vi "Flow and Pressure Sensor V6.vi"() -> ()   [LabVIEW 2018]
uses:
  <vilib>/Utility/config.llb/Config Data RefNum.ctl
  <vilib>/Utility/sysdir.llb/System Directory Type.ctl
  Program Files/National Instruments/LabVIEW 2018/examples/Instrument IO/Serial/support/Serial - XON-XOFF Characters.ctl
  Program Files/National Instruments/LabVIEW 2018/examples/Instrument IO/Serial/support/Serial - ASCII Characters.ctl
  Program Files/National Instruments/LabVIEW 2018/examples/Instrument IO/Serial/support/Serial - Settings.ctl
  <vilib>/Utility/config.llb/Read Key (String).vi
  <vilib>/Utility/config.llb/Write Key (String).vi
  <vilib>/Utility/config.llb/NI_LVConfig.lvlib
panel:
  out "RPM":string
  in  "Pump Speed":dbl(slide) step=1.0 scale=0.0..1023.0 scale format="%#.2f"
  out "Pressure Output":string
  out "Flow Output":string
  out "Raw Data":string
  out "Pressure":dbl(graph)
  out "Flow":dbl(graph)
  out "error out":errorcluster
  out "queue":refnum<queue>
  out "Driver Status":errorcluster
  in  "Marker":string="start_marker"
  out "State":enum16{"Connect", "Acquire", "Standby"}(ring)=enum."Standby"
  in  "S4":dbl[](array[numeric])=[0.0, 0.0, 0.0, 0.0]
  in  "S3":dbl[](array[numeric])=[0.0, 0.0, 0.0, 0.0]
  in  "S2":dbl[](array[numeric])=[0.0, 0.0, 0.0, 0.0]
  in  "S1":dbl[](array[numeric])=[0.0, 0.0, 0.0, 0.0]
  out "System Path":path
  out "dStruct":string[](array[string])
  out "TDMS":refnum<k34>
  in  "Tab Control":enum32{"Connection", "Diagnostic"}(tab)
  in  "Record":bool
  in  "New File":bool
  in  "markerString":string
  in  "Folder":path
  in  "File Name":string="database"
  in  "VISA":refnum<visa-resource-name>="COM4"
  in  "EXIT":bool
  in  "Connect":bool
  in  "add marker":bool
  out "Latency:":dbl
  out "Terminal":string
  in  "Command Terminal":string
  out "Serial Settings:Number of Bytes at Serial Port":u32
  out "Device:":string
  out "Battery Voltage":dbl(slide) scale=3.2..4.2 scale format="%#_2g"
  out "Error Out":errorcluster
  out "Config File":T1
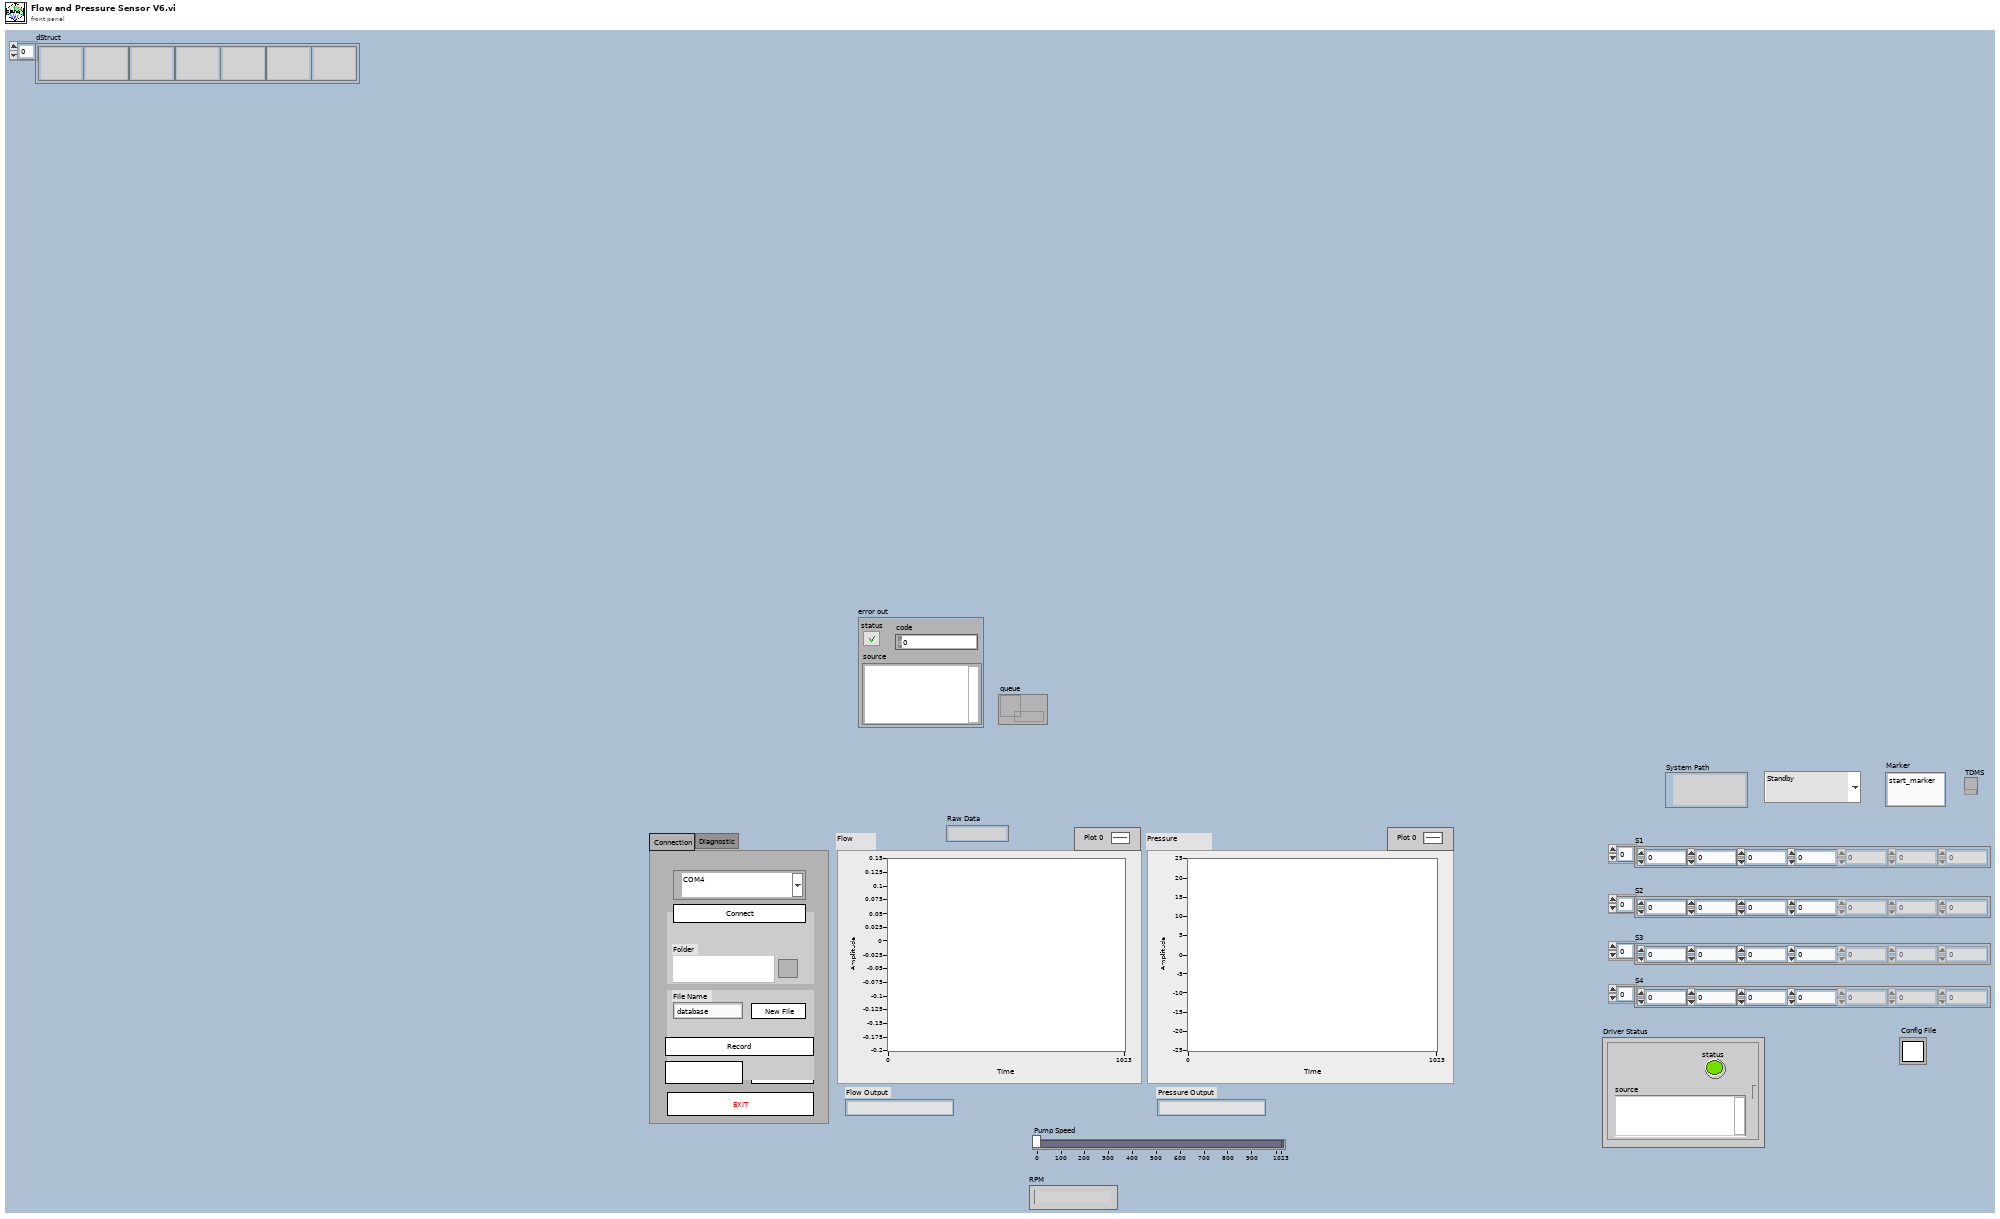
[diagram p1: front panel]
types:
  T1 = typedef "NI_LVConfig.lvlib/Config Data RefNum.ctl" = refnum<k1>
  T2 = cluster{"Dynamic Data Type":dynamicdata, string[]}
  T3 = typedef "System Directory Type.ctl" = i32
  T4 = typedef "Serial - Settings.ctl" = cluster{"baud rate":u32, "data bits":u16, "parity":enum16{"None", "Odd", "Even", "Mark", "Space"}, "stop bits":u16, "flow control":u16}
  T5 = typedef "Serial - XON-XOFF Characters.ctl" = cluster{"XON":T6, "XOFF":T6}
  T6 = typedef "Serial - ASCII Characters.ctl" = enum16{"NUL", "SOH", "STX", "ETX", "EOT", "ENQ", "ACK", "BEL", "BS", "HT", "LF", "VT", "FF", "CR", "SO", "SI", "DLE", "DC1", "DC2", "DC3", "DC4", "NAK", "SYN", "ETB", "CAN", "EM", "SUB", "ESC", "FS", "GS", "RS", "US", "SP", "!", "\"", "#", "$", "%", "&", "'", "(", ")", "*", "+", ",", "- (-)", ".", "/", "0", "1", "2", "3", "4", "5", "6", "7", "8", "9", ":", ";", "<", "=", ">", "?", "@", "A", "B", "C", "D", "E", "F", "G", "H", "I", "J", "K", "L", "M", "N", "O", "P", "Q", "R", "S", "T", "U", "V", "W", "X", "Y", "Z", "[", "\\", "]", "^", "_", "`", "a", "b", "c", "d", "e", "f", "g", "h", "i", "j", "k", "l", "m", "n", "o", "p", "q", "r", "s", "t", "u", "v", "w", "x", "y", "z", "{", "|", "}", "~"}
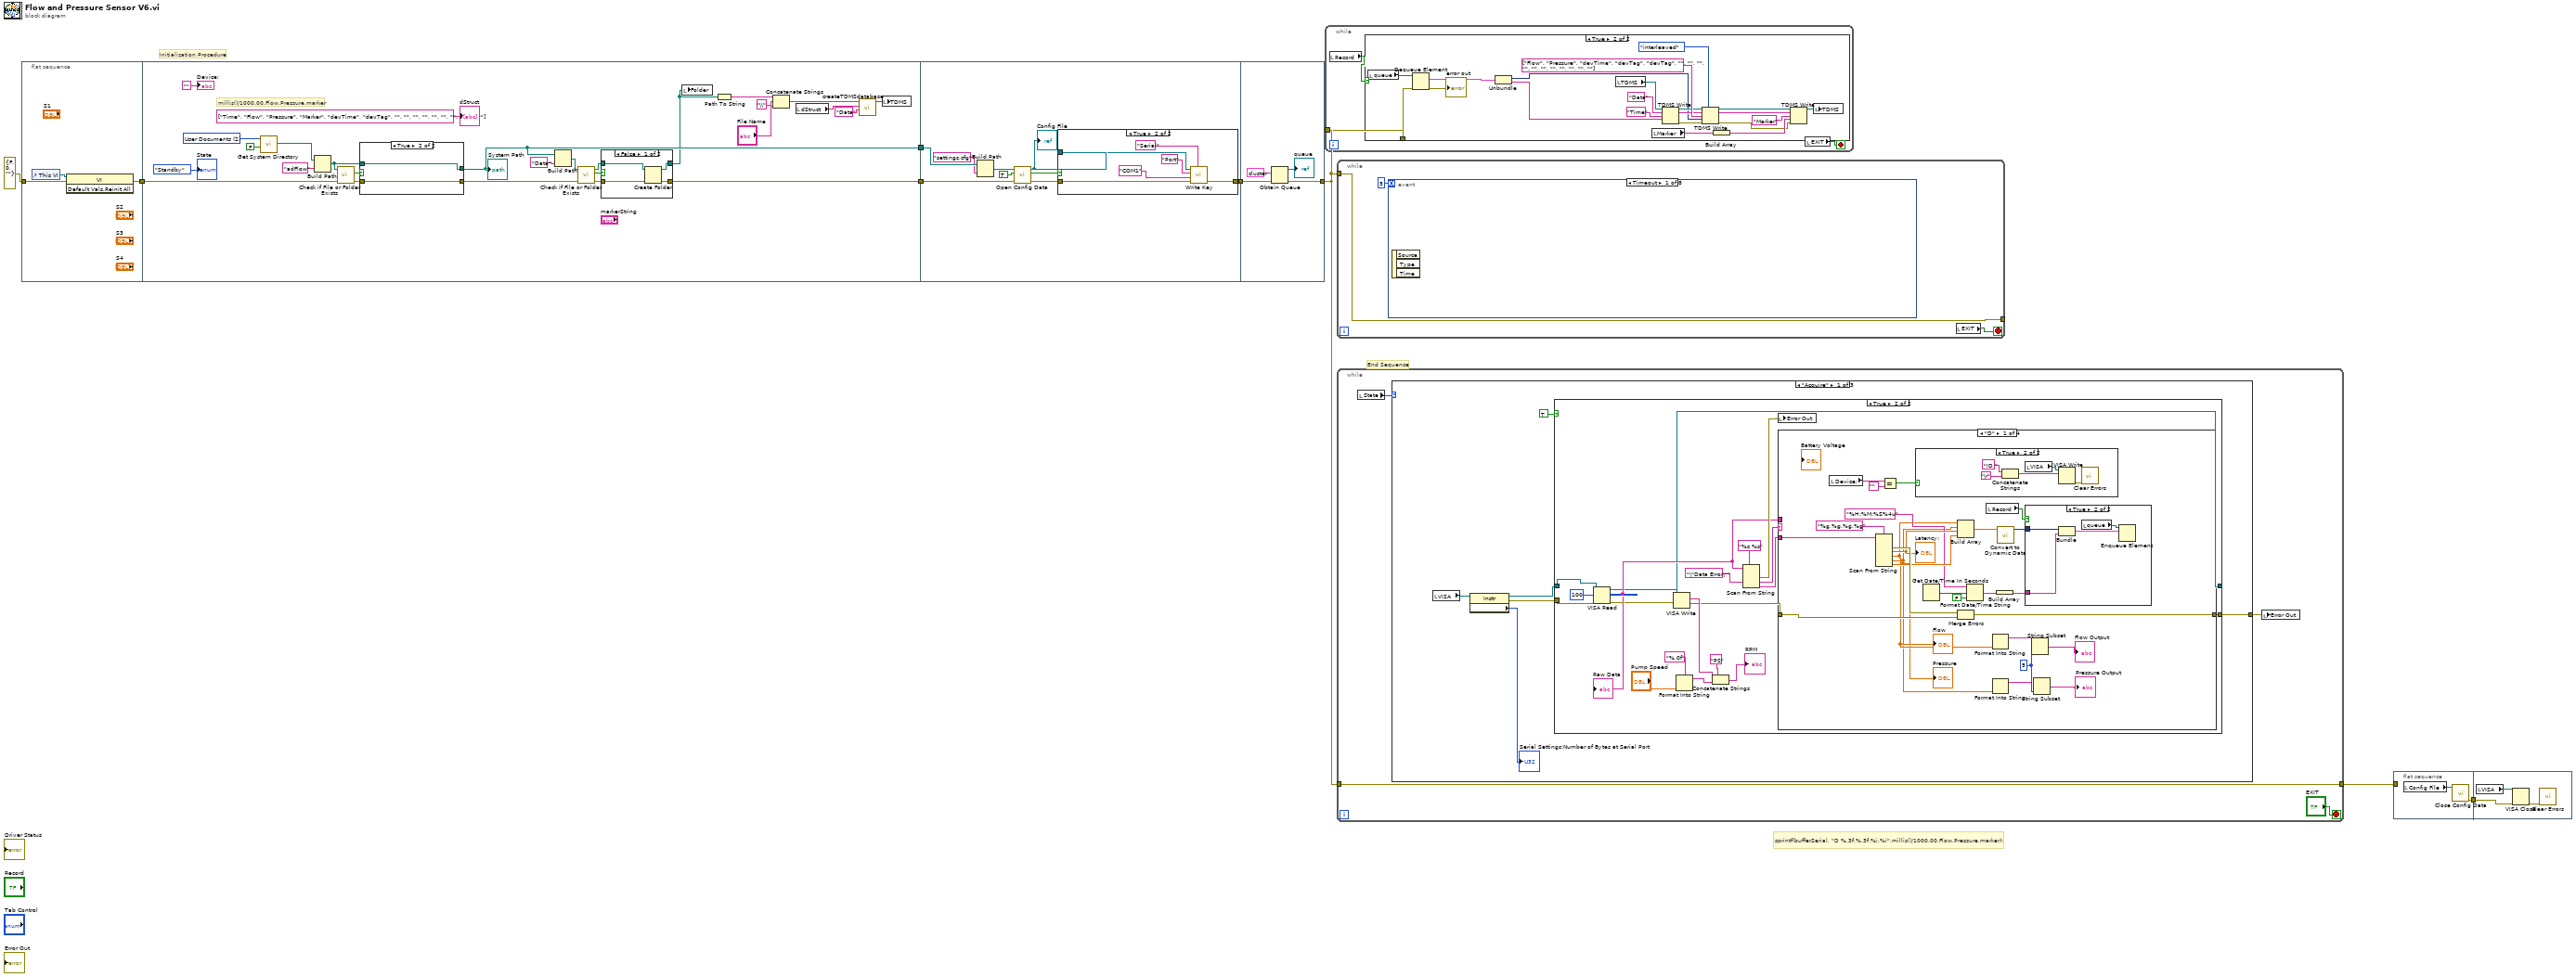
[diagram p0: block diagram]
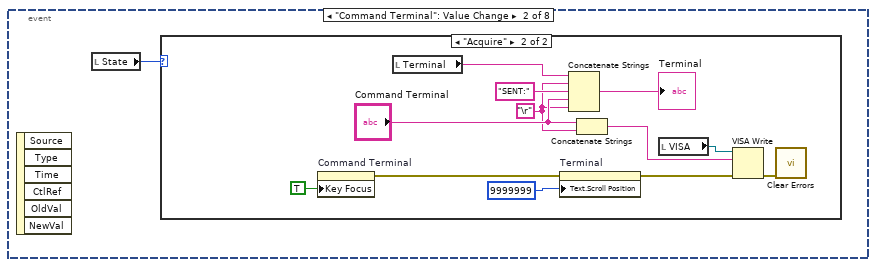
[diagram p3: hidden frame]
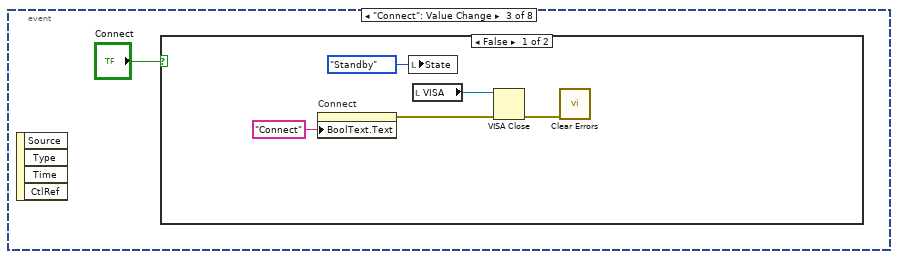
[diagram p5: hidden frame]
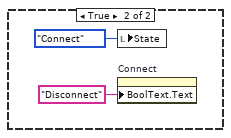
[diagram p6: hidden frame]
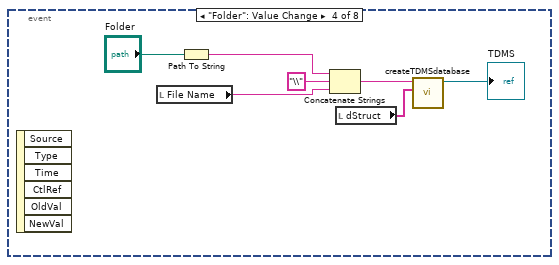
[diagram p7: hidden frame]
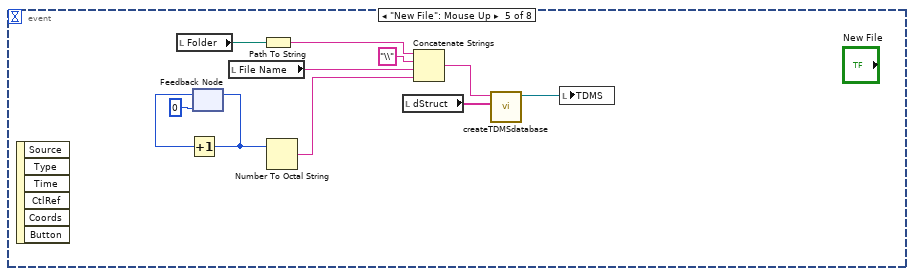
[diagram p8: hidden frame]
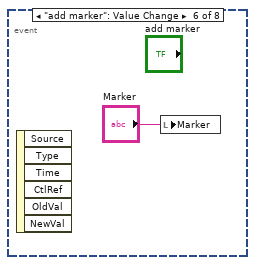
[diagram p9: hidden frame]
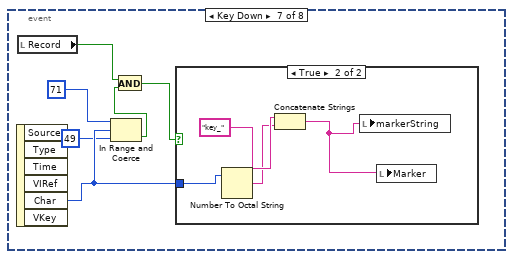
[diagram p10: hidden frame]
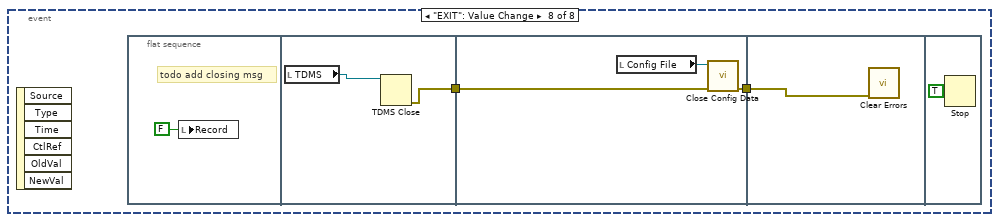
[diagram p12: hidden frame]
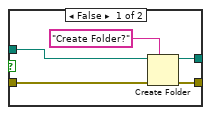
[diagram p14: hidden frame]
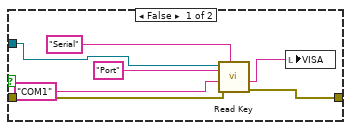
[diagram p15: hidden frame]
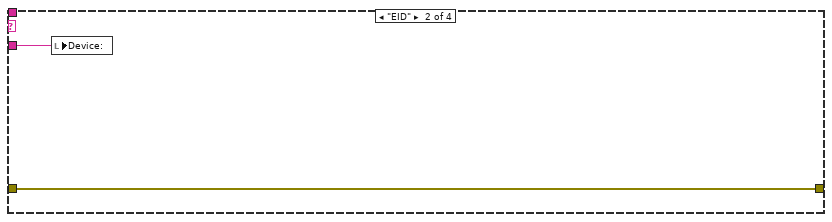
[diagram p19: hidden frame]
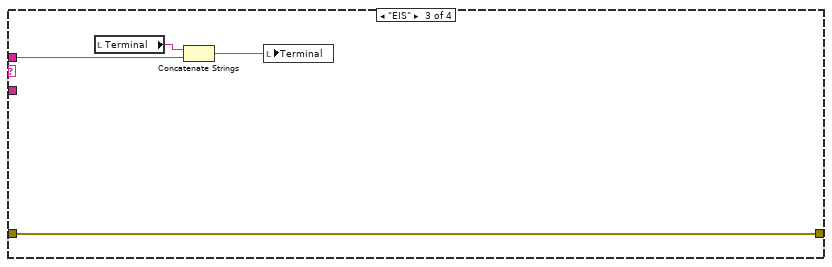
[diagram p20: hidden frame]
diagram:
  # "sprintf(bufferSerial, \"D %.3f,%.3f,%i,%i\",millis()/1000.00,Flow,Pressure,marker);"
  # "End Sequence"
  # "Initialization Procedure"
  n1 = flat-sequence {
    tunnel: errorcluster {"status"=FALSE, "code"=0, "source"=""} ("error in (no error)") -> [w10]
    tunnel: [w9] -> w5
    tunnel: [w28] -> w7
    tunnel: [w25] -> w6
    tunnel: w5 -> [w34]
    tunnel: w7 -> [w58]
    tunnel: w6 -> [w60]
    tunnel: [w52] -> w3
    tunnel: [w75] -> w2
    tunnel: w3 -> [w77]
    frame #0 {
      n2 = control-ref of="This VI"() -> (w11:refnum<vi>)
      n3 = invoke class="VI" method="Default Vals.Reinit All"(reference=w11, error in=w10) -> (error out=w9:errorcluster)  [unwired: 1 in, 2 out]
    }
    frame #1 {
      w37 = T3 2 items=["User Home"=0, "User Desktop"=1, "User Documents"=2, "User Application Data"=3, "User Preferences"=4, "User Temporary"=5, "Public Documents"=6, "Public Application Data"=7, "Public Preferences"=8, "Public Cache"=13, "System Core Libraries"=9, "System Installed Libraries"=10, "Application Files"=11, "Boot Volume Root"=12] ("system directory type")
      # "millis()/1000.00,Flow,Pressure,marker"
      n4 = call <vilib>:"Get System Directory.vi"("create directory if not found? (F)"=FALSE, "system directory type"=w37) -> ("system directory"=w36:path)  [unwired: 9 in]
      n5 = Build Path(base path=w36, name or relative path="adFlow") -> (appended path=w32:path)
      n6 = call <vilib>:"Check if File or Folder Exists.vi"("error in (no error)"=w34, "path"=w32) -> ("error out"=w31:errorcluster, "file or folder exists?"=w33:bool)  [unwired: 7 in, 1 out]
      n7 = case shown="True" w33 {
        tunnel: w32 -> [w49 w51]
        tunnel: w31 -> [w48 w50]
        tunnel: [w46 w51] -> w28
        tunnel: [w45 w50] -> w27
        frame False {
          n8 = Create Folder(prompt (Create Folder)="Create Folder?", path (use dialog)=w49, error in=w48) -> (created path=w46:path, error out=w45:errorcluster)  [unwired: 1 out]
        }
        frame True {
        }
      }
      "System Path" <- w28
      n9 = Build Path(base path=w28, name or relative path="Data") -> (appended path=w29:path)
      n10 = call <vilib>:"Check if File or Folder Exists.vi"("error in (no error)"=w27, "path"=w29) -> ("error out"=w26:errorcluster, "file or folder exists?"=w24:bool, "dup path"=w23:path)  [unwired: 7 in]
      n11 = case shown="False" w24 {
        tunnel: [w41 w44] -> w25
        tunnel: w26 -> [w42 w44]
        tunnel: w23 -> [w40 w43]
        tunnel: [w39 w43] -> w21
        frame False {
          n12 = Create Folder(path (use dialog)=w40, error in=w42) -> (created path=w39:path, error out=w41:errorcluster)  [unwired: 1 in, 1 out]
        }
        frame True {
        }
      }
      n13 = local write "Folder"(w21) -> ()
      n14 = Path To String(path=w21) -> (string=w16:string)
      n15 = Concatenate Strings(w16, "\\" ("string"), "File Name") -> (w20:string)
      n16 = local read "dStruct"() -> (w19:string[])
      n17 = call "createTDMSdatabase.vi"("group name in (Untitled)"="Data", "channel name(s) in (Untitled)"=w19, "String"=w20) -> ("Refnum out"=w22:refnum<k34>)  [unwired: 8 in]
      n18 = local write "TDMS"(w22) -> ()
      "dStruct" <- string[] ["Time", "Flow", "Pressure", "Marker", "devTime", "devTag", "", "", "", "", "", "", "", "", "", ""] ("Channel Names")
      "Device:" <- ""
      "State" <- enum16{"Connect", "Acquire", "Standby"}."Standby" ("State")
    }
    frame #2 {
      n19 = Build Path(base path=w58, name or relative path="settings.cfg") -> (appended path=w56:path)
      n20 = call <vilib>:"Open Config Data.vi"("error in (no error)"=w60, "create file if necessary (T)"=TRUE, "configuration file path"=w56) -> ("error out"=w53:errorcluster, "file created?"=w55:bool, "refnum"=w54:T1)  [unwired: 6 in]
      "Config File" <- w54
      n21 = case shown="True" w55 {
        tunnel: w54 -> [w61 w73]
        tunnel: w53 -> [w63 w72]
        tunnel: [w62 w71] -> w52
        frame False {
          n22 = call-poly <vilib>:"Read Key.vi"("section"="Serial", "error in (no error)"=w63, "default value"="COM1" ("key"), "key"="Port", "refnum"=w61) -> ("error out"=w62:errorcluster, "value"=w67:string)  [unwired: 3 in, 2 out]
          n23 = local write "VISA"(w67) -> ()
        }
        frame True {
          n24 = call-poly <vilib>:"Write Key.vi"("section"="Serial", "error in (no error)"=w72, "value"="COM1" ("key"), "key"="Port", "refnum"=w73) -> ("error out"=w71:errorcluster)  [unwired: 4 in, 2 out]
        }
      }
    }
    frame #3 {
      n25 = Obtain Queue(element data type=T2 {"Dynamic Data Type"=[{"t0"=timestamp(0 s since 1904-01-01), "dt"=1.0, "Y"=[0.0, 0.0, 0.0, 0.0]}, {"t0"=timestamp(3629832558.8844056 s since 1904-01-01), "dt"=1.0, "Y"=[0.0]}, {"t0"=timestamp(3629832558.8844056 s since 1904-01-01), "dt"=1.0, "Y"=[1628.381]}, {"t0"=timestamp(3629832558.8844056 s since 1904-01-01), "dt"=1.0, "Y"=[0.0]}], ["0:00:00.0000"]} ("queue cluster"), error in (no error)=w77) -> (queue out=→"queue":refnum<queue>, error out=w75:errorcluster)  [unwired: 3 in, 1 out]
    }
  }
  n26 = while {
    tunnel: w2 -> [w80]
    stop <- w79 stop-if-true
    n27 = local read "Record"() -> (w78:bool)
    n28 = case shown="True" w78 {
      tunnel: w80 -> [_ w100]
      frame False {
      }
      frame True {
        n29 = local read "queue"() -> (w101:refnum<queue>)
        n30 = Dequeue Element(queue=w101, error in (no error)=w100) -> (element=w99:T2, error out=→"error out":errorcluster)  [unwired: 1 in, 2 out]
        n31 = Unbundle(w99) -> ("Dynamic Data Type"=w83:dynamicdata, w84:string[])
        n32 = local read "TDMS"() -> (w92:refnum<k34>)
        n33 = local read "Marker"() -> (w93:string)
        n34 = TDMS Write(0:w92, 5:"Data" ("group name in (Untitled)"), 7:"Time" ("group name in (Untitled)"), 9:w84) -> (4:w88:refnum<k34>, 6:w89:string, 15:w90:errorcluster)  [unwired: 2 in, 1 out]
        n35 = TDMS Write(0:w88, 1:enum16{"decimated", "interleaved"}."interleaved" ("data layout (0:decimated)"), 5:w89, 7:string[] ["Flow", "Pressure", "devTime", "devTag", "devTag", "", "", "", "", "", "", "", "", "", "", ""] ("Channel Names"), 9:w83, 11:w90) -> (4:w86:refnum<k34>, 6:w85:string, 15:w81:errorcluster)  [unwired: 1 out]
        n36 = Build Array(w93) -> (w94:string[])
        n37 = TDMS Write(0:w86, 5:w85, 7:"Marker" ("channel name(s) in (Untitled)"), 9:w94, 11:w81) -> (4:w97:refnum<k34>)  [unwired: 1 in, 3 out]
        n38 = local write "TDMS"(w97) -> ()
      }
    }
    n39 = local read "EXIT"() -> (w79:bool)
  }
  n40 = while {
    tunnel: w2 -> [w103]
    tunnel: [w103] -> _
    stop <- w104 stop-if-true
    n41 = event shown="[0] Timeout" {
      selector: _ -> [_ _ _ _ _ _ _ _]
      dyn-events: _ -> [_ _ _ _ _ _ _ _]
      timeout: 5 -> [_ _ _ _ _ _ _ _]
      event Timeout {
        n42 = event-data() -> ()  [unwired: 1 in, 3 out]
      }
      event "Command Terminal": Value Change {
        n43 = event-data() -> ()  [unwired: 1 in, 6 out]
        n44 = local read "State"() -> (w105:enum16{"Connect", "Acquire", "Standby"})
        n45 = case shown="\"Acquire\"" w105 {
          frame "Connect", Default {
          }
          frame "Acquire" {
            w108 = "\r"
            n46 = property on="Command Terminal" class="Str"("Key Focus"=TRUE) -> (error out=w113:errorcluster)  [unwired: 2 in, 1 out]
            n47 = local read "Terminal"() -> (w117:string)
            n48 = property on="Terminal" class="Str"(error in=w113, "Text.Scroll Position"=u32 9999999) -> (error out=w109:errorcluster)  [unwired: 1 in, 1 out]
            n49 = Concatenate Strings(w117, w108, "SENT:" ("string"), "Command Terminal", w108) -> (→"Terminal":string)
            n50 = Concatenate Strings("Command Terminal", w108) -> (w110:string)
            n51 = local read "VISA"() -> (w107:refnum<visa-resource-name>)
            n52 = VISA Write(VISA resource name=w107, write buffer=w110, error in (no error)=w109) -> (error out=w106:errorcluster)  [unwired: 2 out]
            n53 = call <vilib>:"Clear Errors.vi"("error in (no error)"=w106) -> ()  [unwired: 5 in, 2 out]
          }
        }
      }
      event "Connect": Value Change {
        n54 = event-data() -> ()  [unwired: 1 in, 4 out]
        n55 = case shown="False" "Connect" {
          frame False {
            n56 = property on="Connect" class="Bool (strict)"("BoolText.Text"="Connect" ("Boolean Text.Text")) -> (error out=w121:errorcluster)  [unwired: 2 in, 1 out]
            n57 = local write "State"(enum16{"Connect", "Acquire", "Standby"}."Standby" ("Enum")) -> ()
            n58 = local read "VISA"() -> (w120:refnum<visa-resource-name>)
            n59 = VISA Close(VISA resource name=w120, error in (no error)=w121) -> (error out=w119:errorcluster)
            n60 = call <vilib>:"Clear Errors.vi"("error in (no error)"=w119) -> ()  [unwired: 5 in, 2 out]
          }
          frame True {
            n61 = local write "State"(enum16{"Connect", "Acquire", "Standby"}."Connect" ("Enum")) -> ()
            n62 = property on="Connect" class="Bool (strict)"("BoolText.Text"="Disconnect" ("Boolean Text.Text")) -> ()  [unwired: 2 in, 2 out]
          }
        }
      }
      event "Folder": Value Change {
        n63 = event-data() -> ()  [unwired: 1 in, 6 out]
        n64 = local read "File Name"() -> (w127:string)
        n65 = Path To String(path="Folder") -> (string=w129:string)
        n66 = Concatenate Strings(w129, "\\" ("string"), w127) -> (w126:string)
        n67 = local read "dStruct"() -> (w130:string[])
        n68 = call "createTDMSdatabase.vi"("channel name(s) in (Untitled)"=w130, "String"=w126) -> ("Refnum out"=→"TDMS":refnum<k34>)  [unwired: 9 in]
      }
      event "New File": Mouse Up {
        n69 = event-data() -> ()  [unwired: 1 in, 6 out]
        n70 = local read "Folder"() -> (w140:path)
        n71 = feedback #1(0) -> (w141:i32)
        n72 = Increment(x=w141) -> (x+1=w143:i32)
        n73 = feedback-in #1(w143) -> ()
        n74 = local read "File Name"() -> (w134:string)
        n75 = Path To String(path=w140) -> (string=w136:string)
        n76 = Number To Octal String(2:w143) -> (0:w133:string)  [unwired: 1 in]
        n77 = local read "dStruct"() -> (w137:string[])
        n78 = Concatenate Strings(w136, "\\" ("string"), w134, w133) -> (w139:string)
        n79 = call "createTDMSdatabase.vi"("channel name(s) in (Untitled)"=w137, "String"=w139) -> ("Refnum out"=w138:refnum<k34>)  [unwired: 9 in]
        n80 = local write "TDMS"(w138) -> ()
      }
      event "add marker": Value Change {
        n81 = event-data() -> ()  [unwired: 1 in, 6 out]
        n82 = local write "Marker"("Marker") -> ()
      }
      event Key Down {
        n83 = event-data() -> ("Char"=w150:i16)  [unwired: 1 in, 5 out]
        n84 = local read "Record"() -> (w148:bool)
        n85 = In Range and Coerce(upper limit=i16 71, x=w150, lower limit=i16 49) -> (In Range?=w146:bool)  [unwired: 1 out]
        n86 = And(x=w148, y=w146) -> (x .and. y?=w145:bool)
        n87 = case shown="True" w145 {
          tunnel: w150 -> [_ w151]
          frame False {
          }
          frame True {
            n88 = Number To Octal String(2:w151) -> (0:w153:string)  [unwired: 1 in]
            n89 = Concatenate Strings("key_" ("element"), w153) -> (w152:string)
            n90 = local write "markerString"(w152) -> ()
            n91 = local write "Marker"(w152) -> ()
          }
        }
      }
      event "EXIT": Value Change {
        n92 = event-data() -> ()  [unwired: 1 in, 6 out]
        n93 = flat-sequence {
          tunnel: [w158] -> w155
          tunnel: [w161] -> w156
          tunnel: w155 -> [w160]
          tunnel: w156 -> [w163]
          frame #0 {
            # "todo add closing msg"
            n94 = local write "Record"(FALSE ("Record")) -> ()
          }
          frame #1 {
            n95 = local read "TDMS"() -> (w159:refnum<k34>)
            n96 = TDMS Close(11:w159) -> (0:w158:errorcluster)  [unwired: 1 in, 1 out]
          }
          frame #2 {
            n97 = local read "Config File"() -> (w162:T1)
            n98 = call <vilib>:"Close Config Data.vi"("error in (no error)"=w160, "refnum"=w162) -> ("error out"=w161:errorcluster)  [unwired: 8 in, 1 out]
          }
          frame #3 {
            n99 = call <vilib>:"Clear Errors.vi"("error in (no error)"=w163) -> ()  [unwired: 5 in, 2 out]
          }
          frame #4 {
            n100 = Stop(stop? (T)=TRUE) -> ()
          }
        }
      }
    }
    n101 = local read "EXIT"() -> (w104:bool)
  }
  n102 = while {
    tunnel: w2 -> [w167]
    tunnel: [w167] -> w4
    stop <- "EXIT" stop-if-true
    n103 = local read "State"() -> (w166:enum16{"Connect", "Acquire", "Standby"})
    n104 = case shown="\"Acquire\"" w166 {
      tunnel: [w174 errorcluster {"status"=FALSE, "code"=0, "source"=""} ("error out") w239] -> w165
      frame "Acquire" {
        n105 = local read "VISA"() -> (w170:refnum<visa-resource-name>)
        n106 = property class="Instr"(reference=w170) -> (reference out=w172:refnum<visa-resource-name>, error out=w173:errorcluster, "Serial Settings:Number of Bytes at Serial Port"=→"Serial Settings:Number of Bytes at Serial Port":u32)  [unwired: 1 in]
        n107 = case shown="True" TRUE {
          tunnel: [w176 w194] -> w174
          tunnel: w173 -> [w176 w181]
          tunnel: w172 -> [w175 w182]
          tunnel: [w175 w179] -> _
          frame False {
          }
          frame True {
            n108 = VISA Read(VISA resource name=w182, byte count=u32 100, error in (no error)=w181) -> (VISA resource name out=w180:refnum<visa-resource-name>, read buffer=w188:string, error out=w177:errorcluster)  [unwired: 1 out]
            "Raw Data" <- w188
            n109 = Format Into String(format string="%.0f", "Pump Speed") -> (resulting string=w186:string)  [unwired: 2 in, 1 out]
            n110 = Concatenate Strings("PS", w186) -> (w187:string)
            "RPM" <- w187
            n111 = VISA Write(VISA resource name=w180, write buffer=w187, error in (no error)=w177) -> (VISA resource name out=w179:refnum<visa-resource-name>, error out=w178:errorcluster)  [unwired: 1 out]
            n112 = Scan From String(format string="%s %s", input string=w188, default 1="\"Data Error\"" ("default value 1")) -> (error out=w190:errorcluster, output 1=w191:string, output 2=w189:string)  [unwired: 3 in, 2 out]
            n113 = local write "Error Out"(w190) -> ()
            n114 = case shown="\"D\"" w191 {
              tunnel: w178 -> [w219 w231 w233 w236]
              tunnel: [w217 w231 w233 w236] -> w194
              tunnel: w188 -> [_ _ w232 _]
              tunnel: w189 -> [w209 w230 _ _]
              frame "D" {
                w201 = u32 5 ("byte count")
                n115 = local read "Device:"() -> (w214:string)
                n116 = Scan From String(format string="%g,%g,%g,%g", input string=w209) -> (error out=w218:errorcluster, output 1=w208:dbl, output 2=w197:dbl, output 3=w196:dbl, output 4=w211:dbl)  [unwired: 6 in, 2 out]
                "Latency:" <- w208
                "Flow" <- w197
                "Pressure" <- w196
                n117 = Equal?(x=w214, y="") -> (x = y?=w213:bool)
                n118 = case shown="True" w213 {
                  frame False {
                  }
                  frame True {
                    n119 = Concatenate Strings("ID " ("string"), "\r") -> (w225:string)
                    n120 = local read "VISA"() -> (w222:refnum<visa-resource-name>)
                    n121 = VISA Write(VISA resource name=w222, write buffer=w225) -> (error out=w221:errorcluster)  [unwired: 1 in, 2 out]
                    n122 = call <vilib>:"Clear Errors.vi"("error in (no error)"=w221) -> ()  [unwired: 5 in, 2 out]
                  }
                }
                n123 = Get Date/Time In Seconds() -> (seconds since 1Jan1904=w206:timestamp)
                n124 = Build Array(w197, w196, w208, w211) -> (w215:dbl[])
                n125 = Merge Errors(w218, w219) -> (w217:errorcluster)
                n126 = Format Date/Time String(time format string (%c)="%H:%M:%S%4u", seconds (now)=w206, UTC format=FALSE) -> (date/time string=w205:string)
                n127 = local read "Record"() -> (w216:bool)
                n128 = Format Into String(w197) -> (resulting string=w202:string)  [unwired: 3 in, 1 out]
                n129 = Format Into String(w196) -> (resulting string=w200:string)  [unwired: 3 in, 1 out]
                n130 = Build Array(w205) -> (w203:string[])
                n131 = call "Convert to Dynamic Data"("Array"=w215) -> ("Dynamic Data Type"=w210:dynamicdata)  [unwired: 3 in]
                n132 = case shown="True" w216 {
                  tunnel: w210 -> [_ w229]
                  tunnel: w203 -> [_ w228]
                  frame False {
                  }
                  frame True {
                    n133 = Bundle("Dynamic Data Type"=w229, w228) -> (w227:T2)  [unwired: 1 in]
                    n134 = local read "queue"() -> (w226:refnum<queue>)
                    n135 = Enqueue Element(queue=w226, element=w227) -> ()  [unwired: 2 in, 3 out]
                  }
                }
                n136 = String Subset(string=w202, length (rest)=w201) -> (substring=→"Flow Output":string)  [unwired: 1 in]
                n137 = String Subset(string=w200, length (rest)=w201) -> (substring=→"Pressure Output":string)  [unwired: 1 in]
              }
              frame "EID" {
                n138 = local write "Device:"(w230) -> ()
              }
              frame "EIS" {
                n139 = local read "Terminal"() -> (w234:string)
                n140 = Concatenate Strings(w234, w232) -> (w235:string)
                n141 = local write "Terminal"(w235) -> ()
              }
              frame "Data Error", Default {
              }
            }
          }
        }
      }
      frame "Standby", Default {
      }
      frame "Connect" {
        n142 = call "open_serial.vi"("End Write on Termination Character?"=TRUE, "XON/XOFF Characters"=T5 {"XON"=enum."DC1", "XOFF"=enum."DC3"}, "Termination Character"=u8 10, "Serial Settings"=T4 {"baud rate"=9600, "data bits"=8, "parity"=enum."None", "stop bits"=10, "flow control"=0}, "End Read on Termination Character?"=TRUE, "VISA Refnum in"="VISA") -> ("error out"=w241:errorcluster)  [unwired: 4 in, 1 out]
        n143 = call <vilib>:"Clear Errors.vi"("error in (no error)"=w241) -> ("error out"=w238:errorcluster)  [unwired: 5 in, 1 out]
        n144 = case shown="No Error" w238 {
          selector: w238 -> [w250 w254]
          tunnel: [w249 w254] -> w239
          frame No Error {
            n145 = local read "Config File"() -> (w247:T1)
            n146 = local read "VISA"() -> (w248:refnum<visa-resource-name>)
            n147 = call-poly <vilib>:"Write Key.vi"("section"="Serial", "error in (no error)"=w250, "value"=w248, "key"="Port", "refnum"=w247) -> ("error out"=w249:errorcluster)  [unwired: 4 in, 2 out]
            n148 = local write "State"(enum16{"Connect", "Acquire", "Standby"}."Acquire" ("Enum")) -> ()
          }
          frame Error {
            n149 = local read "VISA"() -> (w256:refnum<visa-resource-name>)
            n150 = property on="Connect" class="Bool (strict)"("Value"=FALSE ("Connect")) -> ()  [unwired: 2 in, 2 out]
            n151 = VISA Close(VISA resource name=w256) -> (error out=w255:errorcluster)  [unwired: 1 in]
            n152 = call <vilib>:"Clear Errors.vi"("error in (no error)"=w255) -> ()  [unwired: 5 in, 2 out]
            n153 = local write "State"(enum16{"Connect", "Acquire", "Standby"}."Standby" ("Enum")) -> ()
          }
        }
      }
    }
    n154 = local write "Error Out"(w165) -> ()
  }
  n155 = flat-sequence {
    tunnel: w4 -> [_]
    tunnel: [w259] -> w1
    tunnel: w1 -> [w261]
    frame #0 {
      n156 = local read "Config File"() -> (w260:T1)
      n157 = call <vilib>:"Close Config Data.vi"("refnum"=w260) -> ("error out"=w259:errorcluster)  [unwired: 9 in, 1 out]
    }
    frame #1 {
      n158 = local read "VISA"() -> (w262:refnum<visa-resource-name>)
      n159 = VISA Close(VISA resource name=w262, error in (no error)=w261) -> (error out=w263:errorcluster)
      n160 = call <vilib>:"Clear Errors.vi"("error in (no error)"=w263) -> ()  [unwired: 5 in, 2 out]
    }
  }
